vi "svfa_Process FRF.vi"(0 "stimulus signal X [EUx]":waveform(dbl), 1 "response signal Y [EUy]":waveform(dbl), 2 "window":T9=1 items=["None"=0, "Hanning"=1, "Hamming"=2, "Blackman-Harris"=3, "Exact Blackman"=4, "Blackman"=5, "Flat Top"=6, "4 Term B-Harris "=7, "7 Term B-Harris"=8, "Low Sidelobe"=9, "Force - Exponential"=10, "Blackman Nuttall"=11, "Triangle"=30, "Bartlett-Hanning"=31, "Bohman"=32, "Parzen"=33, "Welch"=34, "Kaiser"=60, "Dolph-Chebyshev"=61, "Gaussian"=62], 3 "force/exp settings":T8={"force window [%]"=50.0, "exp window [%]"=10.0} {"exp window [%]" min=0.0 max=100.0 format="%.2f"; "force window [%]" min=0.0 max=100.0 format="%.2f"}, 4 "averaging parameters":T11={"averaging mode"=enum."No averaging", "weighting mode"=enum."Linear", "number of averages"=10, "linear mode"=enum."Auto restart"}, 5 "error in (no error)":errorcluster, 7 "processing control":T10(ring), 9 "FRF mode":enum16{"H1", "H2", "H3"}(ring), 11 "spectrum info in":T1 {"x-axis units" items=["Time (s)"=0, "Frequency-CB (Hz)"=1, "Frequency-CPB (Hz)"=1248, "Frequency-Arbitrary (Hz)"=2357, "Quefrency (s)"=2, "Revolutions (rev)"=3, "Order"=4, "Speed (RPM)"=11, "Speed (rad/s)"=21, "Index"=65535]; "weighting filter" items=["Linear", "A-weighting", "B-weighting", "C-weighting", "ITU-R 468-4", "Dolby", "CCITT", "C-message", "Wb", "Wc", "Wd", "We", "Wf", "Wh", "Wj", "Wk", "Wm", "AES17 20 kHz lowpass", "AES17 40 kHz lowpass", "AES17 20 kHz highpass", "AES17 40 kHz highpass"]; "dB reference [EU]" format="%.2f"; "engineering units" items=["custom..."=0, "V"=1, "A"=21, "C"=30, "pC"=31, "s"=32, "-"=29, "Pa"=2, "N"=20, "g"=3, "m/s^2"=4, "m/s"=5, "m"=6, "mm/s"=12, "mm"=13, "micron/s"=14, "micron"=15, "in/s^2"=7, "in/s"=8, "in"=9, "mil/s"=10, "mil"=11, "rad/s^2"=16, "rad/s"=17, "rad"=18, "deg/s^2"=26, "deg/s"=27, "deg"=28, "RPM"=22, "cycle/s^2"=23, "Hz"=24, "cycle"=25, "strain"=19]; "spectral info"."window" items=["None "=0, "Hanning"=1, "Hamming"=2, "Blackman-Harris"=3, "Exact Blackman"=4, "Blackman"=5, "Flat Top"=6, "4 Term B-Harris "=7, "7 Term B-Harris"=8, "Low Sidelobe"=9, "Force - Exponential"=10, "Gaussian"=62]}) -> (8 "stimulus signal X [EUx]":waveform(dbl), 10 "response signal Y [EUy]":waveform(dbl), 12 "averages completed":dbl format="%.2f", 13 "processing control":T10(ring), 14 "complex frequency response":T7={"f0"=0.0, "df"=1.0, "complex spectrum"=[]} {"complex spectrum" format="%.2f"; "df" format="%.2f"; "f0" format="%.2f"}, 16 "coherence":cluster{"f0":dbl, "df":dbl, "coherence":dbl[]} {"coherence" format="%.2f"; "df" format="%.2f"; "f0" format="%.2f"}, 17 "averaging done":bool, 18 "spectrum info out":T1={"channel name"="", "description"="", "x-axis units"=0, "spectral info"={"spectrum type"=enum."Power [Magnitude^2]", "linear/dB"=enum."linear", "window"=0, "window size"=0, "FFT size"=0}, "engineering units"=0, "custom label"="", "dB reference [EU]"=0.0, "peak units"=enum."rms", "weighting filter"=0, "spectral density?"=FALSE, "unit label"="", "spectrum skewed?"=FALSE, "complimentary spectrum units"=enum."none"} {"x-axis units" items=["Time (s)"=0, "Frequency-CB (Hz)"=1, "Frequency-CPB (Hz)"=1248, "Frequency-Arbitrary (Hz)"=2357, "Quefrency (s)"=2, "Revolutions (rev)"=3, "Order"=4, "Speed (RPM)"=11, "Speed (rad/s)"=21, "Index"=65535]; "weighting filter" items=["Linear", "A-weighting", "B-weighting", "C-weighting", "ITU-R 468-4", "Dolby", "CCITT", "C-message", "Wb", "Wc", "Wd", "We", "Wf", "Wh", "Wj", "Wk", "Wm", "AES17 20 kHz lowpass", "AES17 40 kHz lowpass", "AES17 20 kHz highpass", "AES17 40 kHz highpass"]; "dB reference [EU]" format="%.2f"; "engineering units" items=["custom..."=0, "V"=1, "A"=21, "C"=30, "pC"=31, "s"=32, "-"=29, "Pa"=2, "N"=20, "g"=3, "m/s^2"=4, "m/s"=5, "m"=6, "mm/s"=12, "mm"=13, "micron/s"=14, "micron"=15, "in/s^2"=7, "in/s"=8, "in"=9, "mil/s"=10, "mil"=11, "rad/s^2"=16, "rad/s"=17, "rad"=18, "deg/s^2"=26, "deg/s"=27, "deg"=28, "RPM"=22, "cycle/s^2"=23, "Hz"=24, "cycle"=25, "strain"=19]; "spectral info"."window" items=["None "=0, "Hanning"=1, "Hamming"=2, "Blackman-Harris"=3, "Exact Blackman"=4, "Blackman"=5, "Flat Top"=6, "4 Term B-Harris "=7, "7 Term B-Harris"=8, "Low Sidelobe"=9, "Force - Exponential"=10, "Gaussian"=62]}, 19 "error out":errorcluster)   [LabVIEW 2017]
uses:
  <vilib>/addons/_NISVFA/_Shared subVIs/Controls/svc_Window [Dual FFT].ctl
  <vilib>/addons/_NISVFA/_Shared subVIs/Controls/svc_Spectrum Info.ctl
  <vilib>/addons/_NISVFA/_Shared subVIs/Controls/svc_X-Axis Units.ctl
  <vilib>/addons/_NISVFA/_Shared subVIs/Controls/svc_Spectrum Type.ctl
  <vilib>/addons/_NISVFA/_Shared subVIs/Controls/svc_Engineering Units Text Ring.ctl
  <vilib>/addons/_NISVFA/_Shared subVIs/Controls/svc_Weighting Filter Text Ring.ctl
  <vilib>/addons/_NISVFA/_Shared subVIs/Controls/svc_Complimentary Spectrum Units.ctl
  <vilib>/addons/_NISVFA/_Shared subVIs/Windowing/svfa_Scaled Time Domain Window (1 Ch).vi
  <vilib>/addons/_NISVFA/_Shared subVIs/Spectrum Averaging/svfa_Average Array (complex).vi
  <vilib>/addons/_NISVFA/_Shared subVIs/Spectrum Averaging/svfa_Average Array (real).vi
  <vilib>/addons/_NISVFA/_Shared subVIs/Windowing/svfa_Scaled Time Domain Window (Array).vi
  <vilib>/Analysis/4window.llb/Force Window.vi
  <vilib>/Analysis/4window.llb/Force Window (DBL).vi
  <vilib>/Analysis/4window.llb/Exponential Window.vi
  <vilib>/Analysis/4window.llb/Exponential Window (DBL).vi
  <vilib>/Utility/error.llb/Error Cluster From Error Code.vi
  <vilib>/Analysis/0measdsp.llb/Scaled Time Domain Window.vi
  <vilib>/Analysis/0measdsp.llb/Scaled Time Domain Window (DBL).vi
  <vilib>/addons/_NISVFA/_Spectrum Processing/subVIs/svfa_Spectrum Info Window to windowTd Type Def.vi
  <vilib>/addons/_NISVFA/_Shared subVIs/Common/svc_Window Parameters.vi
  <vilib>/addons/_NISVFA/_Shared subVIs/Common/svc_Get Window Info.vi
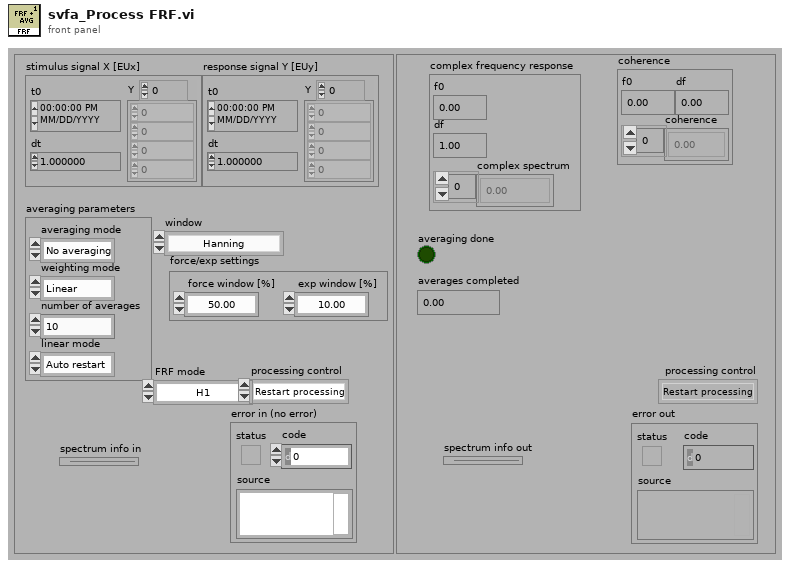
[diagram p1: front panel]
types:
  T1 = typedef "svc_Spectrum Info.ctl" = cluster{"channel name":string, "description":string, "x-axis units":T2, "spectral info":cluster{"spectrum type":T3, "linear/dB":enum16{"linear", "dB"}, "window":u16, "window size":i32, "FFT size":i32}, "engineering units":T4, "custom label":string, "dB reference [EU]":dbl, "peak units":enum16{"rms", "peak", "peak-peak"}, "weighting filter":T5, "spectral density?":bool, "unit label":string, "spectrum skewed?":bool, "complimentary spectrum units":T6}
  T2 = typedef "svc_X-Axis Units.ctl" = u16
  T3 = typedef "svc_Spectrum Type.ctl" = enum16{"FFT Spectrum [complex]", "Amplitude [Magnitude]", "Power [Magnitude^2]", "Cross Spectrum [complex]", "Frequency Response [Complex]"}
  T4 = typedef "svc_Engineering Units Text Ring.ctl" = u16
  T5 = typedef "svc_Weighting Filter Text Ring.ctl" = u16
  T6 = typedef "svc_Complimentary Spectrum Units.ctl" = enum16{"none", "radians", "degrees", "cycles", "imaginary"}
  T7 = cluster{"f0":dbl, "df":dbl, "complex spectrum":cdb[]}
  T8 = cluster{"force window [%]":dbl, "exp window [%]":dbl}
  T9 = typedef "svc_Window [Dual FFT].ctl" = u32
  T10 = enum16{"Restart processing", "Continue processing", "Skip processing"}
  T11 = cluster{"averaging mode":enum16{"No averaging", "Vector averaging", "RMS averaging", "Peak hold"}, "weighting mode":enum16{"Linear", "Exponential"}, "number of averages":u32, "linear mode":enum16{"One shot", "Auto restart"}}
  T12 = enum16{"No averaging", "Vector averaging", "RMS averaging", "Peak hold"}
  T13 = cluster{"f0":dbl, "df":dbl, "complex array":cdb[]}
  T14 = cluster{"complex spectrum":cluster{"f0":dbl, "df":dbl, "complex spectrum":cdb[]}, "spectrum info":T1}
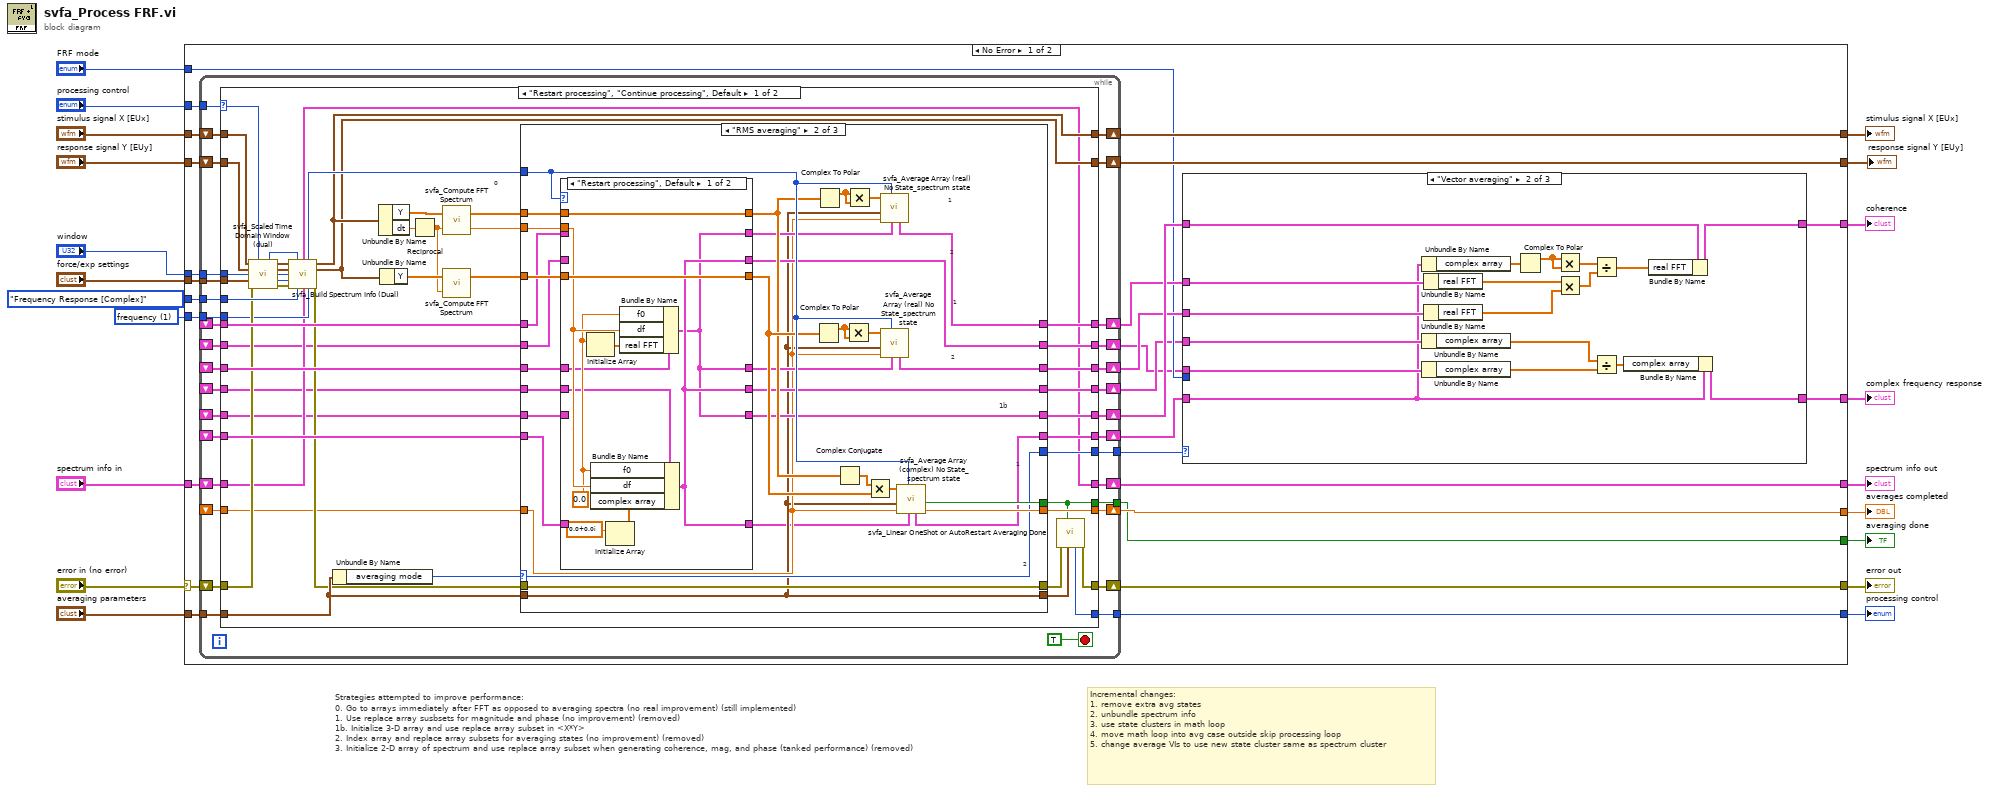
[diagram p0: block diagram]
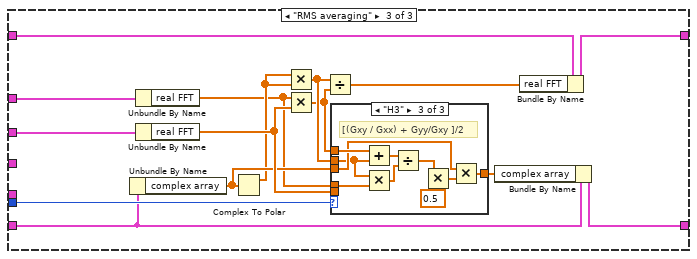
[diagram p3: hidden frame]
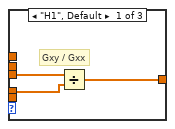
[diagram p4: hidden frame]
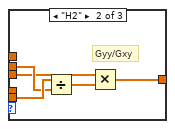
[diagram p5: hidden frame]
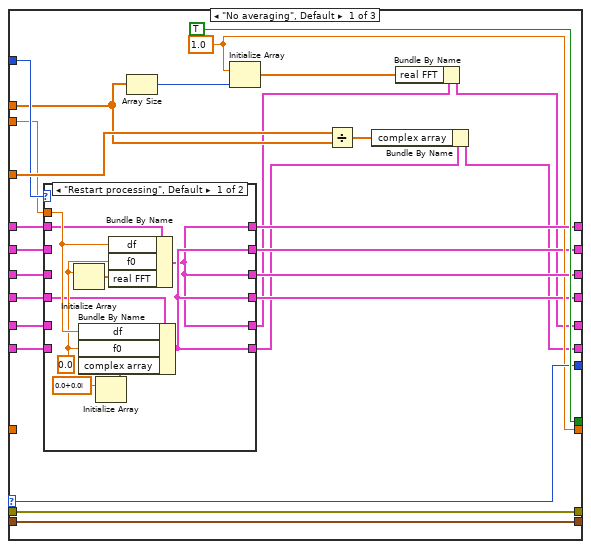
[diagram p6: hidden frame]
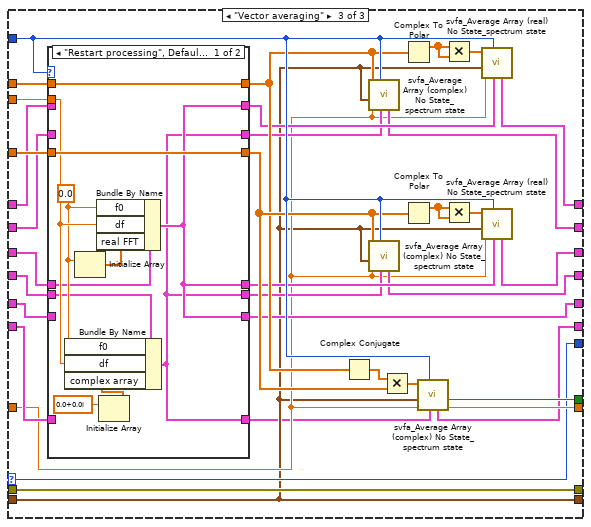
[diagram p9: hidden frame]
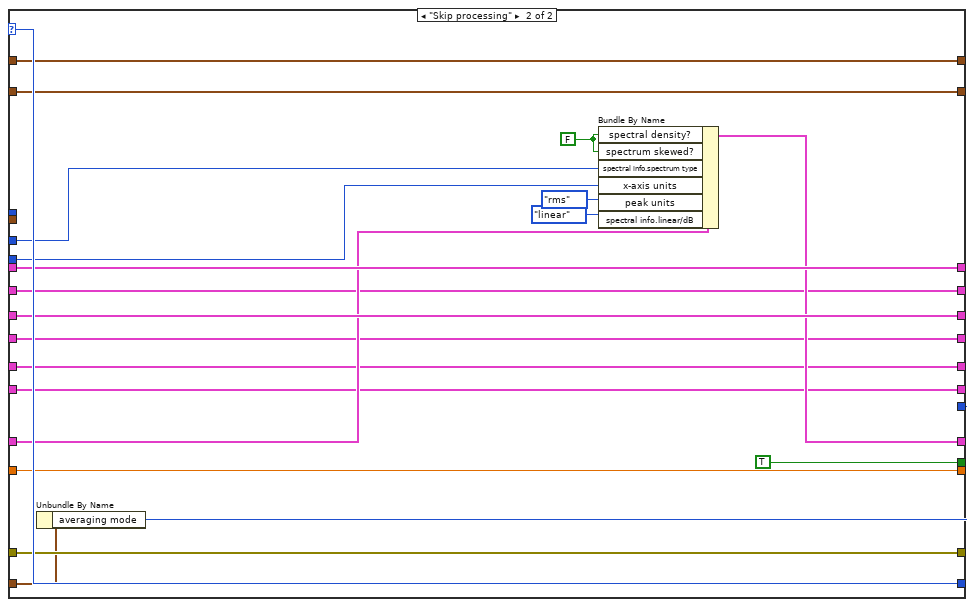
[diagram p11: hidden frame]
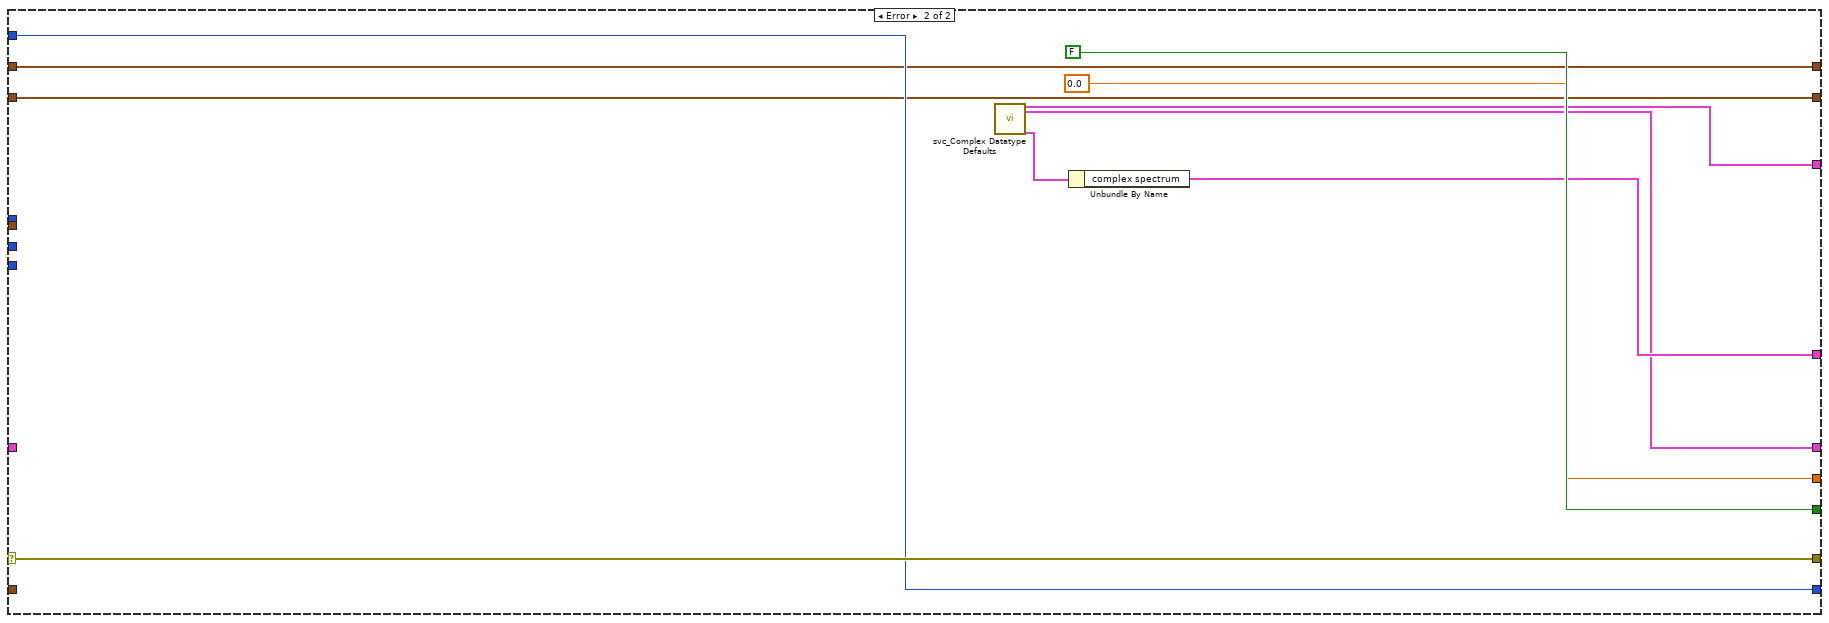
[diagram p12: hidden frame]
diagram:
  w6 = u16 1 items=["time"=0, "frequency"=1, "quefrency"=2, "revolutions"=3, "order"=4, "rpm"=11] ("x-axis units")
  # "Strategies attempted to improve performance:\n0. Go to arrays immediately after FFT as opposed to averaging spectra (no real improvement) (still implemented)\n1. Use replace array susbsets for magnitude and phase (no improvement) (removed)\n1b. Initialize 3-D array and use replace array subset in <X*Y>\n2. Index array and replace array subsets for averaging states (no improvement) (removed)\n3. Initialize 2-D array of spectrum and use replace array subset when generating coherence, mag, and phase (tanked performance) (removed)"
  # "Incremental changes:\n1. remove extra avg states\n2. unbundle spectrum info\n3. use state clusters in math loop\n4. move math loop into avg case outside skip processing loop\n5. change average VIs to use new state cluster same as spectrum cluster"
  n1 = case shown="No Error" "error in (no error)" {
    selector: "error in (no error)" -> [w44 w359]
    tunnel: [w38 w359] -> w20
    tunnel: "averaging parameters" -> [w47 _]
    tunnel: "stimulus signal X [EUx]" -> [w45 w354]
    tunnel: [w32 FALSE ("averaging done")] -> w16
    tunnel: [w46 0.0 ("averages completed")] -> w15
    tunnel: [w22 w352] -> w14
    tunnel: [w23 w350] -> w13
    tunnel: "FRF mode" -> [w26 _]
    tunnel: "processing control" -> [w43 w356]
    tunnel: [w39 w356] -> w10
    tunnel: "response signal Y [EUy]" -> [w42 w353]
    tunnel: "window" -> [w41 _]
    tunnel: "force/exp settings" -> [w40 _]
    tunnel: svc_Spectrum_Type."Frequency Response [Complex]" ("spectrum type") -> [w37 _]
    tunnel: w6 -> [w36 _]
    tunnel: [w35 w351] -> w5
    tunnel: [w34 w354] -> w4
    tunnel: [w33 w353] -> w3
    tunnel: "spectrum info in" -> [w21 _]
    frame No Error {
      n2 = while {
        tunnel: [w124] -> w39
        tunnel: w40 -> [w125]
        tunnel: w41 -> [w126]
        tunnel: w43 -> [w121]
        tunnel: [w130] -> w32
        tunnel: w47 -> [w132]
        shift-right: [w120] -> w28
        shift-left: _ -> [w119]
        shift-right: [w102] -> w31
        shift-left: _ -> [w105]
        shift-right: [w118] -> w29
        shift-left: _ -> [w117]
        tunnel: w37 -> [w116]
        tunnel: w36 -> [w115]
        tunnel: [w112] -> w27
        shift-right: [w111] -> w34
        shift-left: w45 -> [w129]
        shift-right: [w110] -> w33
        shift-left: w42 -> [w127]
        shift-right: [w123] -> w38
        shift-left: w44 -> [w128]
        shift-right: [w113] -> w35
        shift-left: w21 -> [w114]
        shift-right: [w104] -> w24
        shift-left: _ -> [w107]
        shift-right: [w103] -> w25
        shift-left: _ -> [w106]
        shift-right: [w109] -> w30
        shift-left: _ -> [w108]
        shift-right: [w131] -> w46
        shift-left: _ -> [w101]
        stop <- TRUE stop-if-true
        n3 = case shown="\"Restart processing\", \"Continue processing\", Default" w121 {
          selector: w121 -> [w170 w349]
          tunnel: w132 -> [w166 w340]
          tunnel: [w180 w336] -> w131
          tunnel: [w179 TRUE ("averaging done")] -> w130
          tunnel: w128 -> [w152 w347]
          tunnel: w127 -> [w175 w337]
          tunnel: w126 -> [w174 _]
          tunnel: w125 -> [w162 _]
          tunnel: [w171 w349] -> w124
          tunnel: [w167 w347] -> w123
          tunnel: w129 -> [w176 w338]
          tunnel: [w161 w341] -> w109
          tunnel: [w160 w346] -> w120
          tunnel: w108 -> [w159 w341]
          tunnel: w119 -> [w158 w346]
          tunnel: [w157 w345] -> w118
          tunnel: w117 -> [w156 w345]
          tunnel: w116 -> [w155 w329]
          tunnel: w115 -> [w151 w342]
          tunnel: w114 -> [w150 w344]
          tunnel: [w136 w343] -> w113
          tunnel: [w149 w339] -> w112
          tunnel: [w146 w338] -> w111
          tunnel: [w145 w337] -> w110
          tunnel: w107 -> [w144 w335]
          tunnel: w106 -> [w143 w334]
          tunnel: w105 -> [w142 w333]
          tunnel: [w141 w335] -> w104
          tunnel: [w140 w334] -> w103
          tunnel: [w139 w333] -> w102
          tunnel: w101 -> [w138 w336]
          frame "Restart processing", "Continue processing", Default {
            # "0"
            n4 = call <vilib>:"svfa_Scaled Time Domain Window (dual).vi"("Signal in [X]"=w176, "processing control"=w170, "Signal in [Y]"=w175, "window"=w174, "force/exp settings"=w162, "error in (no error)"=w152) -> ("dup processing control"=w169:T10, "Windowed signal [X]"=w178:waveform(dbl), "Windowed signal [Y]"=w177:waveform(dbl), "window"=w173:T9, "window size"=w164:i32, "error out"=w163:errorcluster)  [unwired: 3 in, 1 out]
            n5 = call <vilib>:"svfa_Build Spectrum Info (Dual).vi"("scaled signal  X [EU]"=w178, "processing control"=w169, "scaled signal  Y [EU]"=w177, "window"=w173, "window size"=w164, "error in (no error)"=w163, "spectrum type"=w155, "spectrum info in"=w150, "x-axis units"=w151) -> ("spectrum info out"=w136:T1, "dup processing control"=w168:T10, "dup scaled signal  X [EU]"=w146:waveform(dbl), "dup scaled signal  Y [EU]"=w145:waveform(dbl), "error out"=w147:errorcluster)  [unwired: 2 in]
            n6 = Unbundle By Name(w166) -> ("averaging mode"=w181:T12)
            n7 = Unbundle By Name ("Get Waveform Components")(w146) -> ("Y"=w135:dbl[], "dt"=w134:dbl)
            n8 = Unbundle By Name ("Get Waveform Components")(w145) -> ("Y"=w137:dbl[])
            n9 = Reciprocal(x=w134) -> (1/x=w133:dbl)
            n10 = call <vilib>:"svfa_Compute FFT Spectrum.vi"("sampling frequency [Hz]"=w133, "signal [EU]"=w135) -> ("df [Hz]"=w148:dbl, "FFT spectrum [EUrms]"=w165:cdb[])
            n11 = call <vilib>:"svfa_Compute FFT Spectrum.vi"("sampling frequency [Hz]"=w133, "signal [EU]"=w137) -> ("FFT spectrum [EUrms]"=w154:cdb[])  [unwired: 1 out]
            n12 = case shown="\"RMS averaging\"" w181 {
              selector: w181 -> [w197 w240 w294]
              tunnel: [w205 w239 w293] -> w153
              tunnel: w147 -> [w205 w239 w293]
              tunnel: w166 -> [w206 w231 w283]
              tunnel: [TRUE ("averaging done") w255 w309] -> w179
              tunnel: w168 -> [w203 w253 w307]
              tunnel: [w194 w254 w308] -> w180
              tunnel: [w206 w231 w283] -> w172
              tunnel: w165 -> [w195 w251 w305]
              tunnel: w154 -> [w204 w252 w306]
              tunnel: [w182 w224 w275] -> w161
              tunnel: [w198 w242 w296] -> w160
              tunnel: w159 -> [w200 w246 w301]
              tunnel: w158 -> [w201 w245 w298]
              tunnel: [w199 w243 w297] -> w157
              tunnel: w156 -> [w202 w244 w299]
              tunnel: w148 -> [w196 w241 w295]
              tunnel: [w197 w240 w294] -> w149
              tunnel: w144 -> [w189 w237 w287]
              tunnel: w143 -> [w191 w235 w286]
              tunnel: w142 -> [w192 w233 w285]
              tunnel: [w190 w238 w291] -> w141
              tunnel: [w188 w236 w289] -> w140
              tunnel: [w185 w234 w288] -> w139
              tunnel: w138 -> [_ w232 w284]
              frame "No averaging", Default {
                w194 = 1.0 ("overwrite value")
                n13 = case shown="\"Restart processing\", Default" w203 {
                  tunnel: [w209 w222] -> w199
                  tunnel: w202 -> [w208 w222]
                  tunnel: [w209 w221] -> w198
                  tunnel: w201 -> [_ w221]
                  tunnel: [w210 w220] -> w183
                  tunnel: w200 -> [_ w220]
                  tunnel: w196 -> [w216 _]
                  tunnel: w192 -> [_ w217]
                  tunnel: w191 -> [w211 w218]
                  tunnel: w189 -> [_ w219]
                  tunnel: [w210 w219] -> w190
                  tunnel: [w210 w218] -> w188
                  tunnel: [w209 w217] -> w184
                  frame "Restart processing", Default {
                    w214 = 0.0 ("f0")
                    n14 = Initialize Array(w214) -> (w215:dbl[])  [unwired: 1 in]
                    n15 = Initialize Array(cdb 0.0+0.0i ("element")) -> (w212:cdb[])  [unwired: 1 in]
                    n16 = Bundle By Name(cluster=w211, "df"=w216, "f0"=w214, "complex array"=w212) -> (w210:T13)
                    n17 = Bundle By Name(cluster=w208, "df"=w216, "f0"=w214, "real FFT"=w215) -> (w209:cluster{"f0":dbl, "df":dbl, "real FFT":dbl[]})
                  }
                  frame "Continue processing" {
                  }
                }
                n18 = Array Size(array=w195) -> (size(s)=w186:i32)
                n19 = Initialize Array(w194, w186) -> (w193:dbl[])
                n20 = Divide(x=w204, y=w195) -> (x/y=w187:cdb[])
                n21 = Bundle By Name(cluster=w183, "complex array"=w187) -> (w182:T13)
                n22 = Bundle By Name(cluster=w184, "real FFT"=w193) -> (w185:cluster{"f0":dbl, "df":dbl, "real FFT":dbl[]})
              }
              frame "RMS averaging" {
                # "1"
                # "1b"
                # "2"
                # "2"
                # "2"
                # "1"
                # "1"
                n23 = case shown="\"Restart processing\", Default" w253 {
                  tunnel: w252 -> [w266 w271]
                  tunnel: w251 -> [w264 w274]
                  tunnel: [w266 w271] -> w250
                  tunnel: [w264 w274] -> w249
                  tunnel: [w257 w273] -> w223
                  tunnel: [w256 w272] -> w248
                  tunnel: [w256 w270] -> w247
                  tunnel: w246 -> [_ w273]
                  tunnel: w244 -> [_ w272]
                  tunnel: w245 -> [w259 w270]
                  tunnel: w241 -> [w265 _]
                  tunnel: [w257 w269] -> w238
                  tunnel: w237 -> [_ w269]
                  tunnel: [w257 w268] -> w236
                  tunnel: w235 -> [w258 w268]
                  tunnel: [w256 w267] -> w234
                  tunnel: w233 -> [_ w267]
                  frame "Restart processing", Default {
                    w262 = 0.0 ("f0")
                    n24 = Initialize Array(w262) -> (w263:dbl[])  [unwired: 1 in]
                    n25 = Initialize Array(cdb 0.0+0.0i ("element")) -> (w260:cdb[])  [unwired: 1 in]
                    n26 = Bundle By Name(cluster=w258, "f0"=w262, "df"=w265, "complex array"=w260) -> (w257:T13)
                    n27 = Bundle By Name(cluster=w259, "f0"=w262, "df"=w265, "real FFT"=w263) -> (w256:cluster{"f0":dbl, "df":dbl, "real FFT":dbl[]})
                  }
                  frame "Continue processing", "Skip processing" {
                  }
                }
                n28 = Complex To Polar(r * e^(i*theta)=w250) -> (r=w230:dbl[])  [unwired: 1 out]
                n29 = Complex To Polar(r * e^(i*theta)=w249) -> (r=w228:dbl[])  [unwired: 1 out]
                n30 = Complex Conjugate(1:w249) -> (0:w225:cdb[])
                n31 = Multiply(x=w230, y=w230) -> (x*y=w229:dbl[])
                n32 = Multiply(x=w228, y=w228) -> (x*y=w227:dbl[])
                n33 = Multiply(x=w225, y=w250) -> (x*y=w226:cdb[])
                n34 = call <vilib>:"svfa_Average Array (real) No State_spectrum state.vi"("previous avg real spectrum"=w248, "processing control"=w253, "averages completed"=w232, "averaging parameters"=w231, "array"=w227) -> ("new avg real spectrum"=w243:cluster{"f0":dbl, "df":dbl, "real FFT":dbl[]})  [unwired: 4 in, 2 out]
                n35 = call <vilib>:"svfa_Average Array (real) No State_spectrum state.vi"("previous avg real spectrum"=w247, "processing control"=w253, "averages completed"=w232, "averaging parameters"=w231, "array"=w229) -> ("new avg real spectrum"=w242:cluster{"f0":dbl, "df":dbl, "real FFT":dbl[]})  [unwired: 4 in, 2 out]
                n36 = call <vilib>:"svfa_Average Array (complex) No State_spectrum state.vi"("previous avg complex spectrum"=w223, "processing control"=w253, "averages completed in"=w232, "averaging parameters"=w231, "array"=w226) -> ("averages completed out"=w254:dbl, "averaging done"=w255:bool, "avg complex spectrum"=w224:T13)  [unwired: 4 in]
              }
              frame "Vector averaging" {
                n37 = case shown="\"Restart processing\", Default" w307 {
                  tunnel: w306 -> [w320 w328]
                  tunnel: w305 -> [w318 w327]
                  tunnel: [w320 w328] -> w304
                  tunnel: [w318 w327] -> w303
                  tunnel: [w310 w326] -> w276
                  tunnel: [w311 w325] -> w302
                  tunnel: w301 -> [_ w326]
                  tunnel: w299 -> [_ w325]
                  tunnel: [w311 w324] -> w300
                  tunnel: w298 -> [w313 w324]
                  tunnel: w295 -> [w319 _]
                  tunnel: [w310 w323] -> w292
                  tunnel: [w310 w322] -> w290
                  tunnel: [w311 w321] -> w288
                  tunnel: w287 -> [_ w323]
                  tunnel: w286 -> [w312 w322]
                  tunnel: w285 -> [_ w321]
                  frame "Restart processing", Default {
                    w317 = 0.0 ("f0")
                    n38 = Initialize Array(w317) -> (w316:dbl[])  [unwired: 1 in]
                    n39 = Bundle By Name(cluster=w313, "f0"=w317, "df"=w319, "real FFT"=w316) -> (w311:cluster{"f0":dbl, "df":dbl, "real FFT":dbl[]})
                    n40 = Initialize Array(cdb 0.0+0.0i ("element")) -> (w314:cdb[])  [unwired: 1 in]
                    n41 = Bundle By Name(cluster=w312, "f0"=w317, "df"=w319, "complex array"=w314) -> (w310:T13)
                  }
                  frame "Continue processing", "Skip processing" {
                  }
                }
                n42 = Complex Conjugate(1:w303) -> (0:w278:cdb[])
                n43 = call <vilib>:"svfa_Average Array (complex) No State_spectrum state.vi"("previous avg complex spectrum"=w292, "processing control"=w307, "averages completed in"=w284, "averaging parameters"=w283, "array"=w303) -> ("avg complex spectrum"=w291:T13)  [unwired: 4 in, 2 out]
                n44 = call <vilib>:"svfa_Average Array (complex) No State_spectrum state.vi"("previous avg complex spectrum"=w290, "processing control"=w307, "averages completed in"=w284, "averaging parameters"=w283, "array"=w304) -> ("avg complex spectrum"=w289:T13)  [unwired: 4 in, 2 out]
                n45 = Multiply(x=w278, y=w304) -> (x*y=w277:cdb[])
                n46 = Complex To Polar(r * e^(i*theta)=w303) -> (r=w280:dbl[])  [unwired: 1 out]
                n47 = Complex To Polar(r * e^(i*theta)=w304) -> (r=w282:dbl[])  [unwired: 1 out]
                n48 = call <vilib>:"svfa_Average Array (complex) No State_spectrum state.vi"("previous avg complex spectrum"=w276, "processing control"=w307, "averages completed in"=w284, "averaging parameters"=w283, "array"=w277) -> ("averages completed out"=w308:dbl, "averaging done"=w309:bool, "avg complex spectrum"=w275:T13)  [unwired: 4 in]
                n49 = Multiply(x=w280, y=w280) -> (x*y=w279:dbl[])
                n50 = Multiply(x=w282, y=w282) -> (x*y=w281:dbl[])
                n51 = call <vilib>:"svfa_Average Array (real) No State_spectrum state.vi"("previous avg real spectrum"=w302, "processing control"=w307, "averages completed"=w284, "averaging parameters"=w283, "array"=w279) -> ("new avg real spectrum"=w297:cluster{"f0":dbl, "df":dbl, "real FFT":dbl[]})  [unwired: 4 in, 2 out]
                n52 = call <vilib>:"svfa_Average Array (real) No State_spectrum state.vi"("previous avg real spectrum"=w300, "processing control"=w307, "averages completed"=w284, "averaging parameters"=w283, "array"=w281) -> ("new avg real spectrum"=w296:cluster{"f0":dbl, "df":dbl, "real FFT":dbl[]})  [unwired: 4 in, 2 out]
              }
            }
            n53 = call <vilib>:"svfa_Linear OneShot or AutoRestart Averaging Done.vi"("averaging parameters"=w172, "averaging done"=w179, "error in (no error)"=w153) -> ("error out"=w167:errorcluster, "processing control"=w171:T10)  [unwired: 7 in]
          }
          frame "Skip processing" {
            w331 = FALSE ("spectral density?")
            n54 = Unbundle By Name(w340) -> ("averaging mode"=w339:T12)
            n55 = Bundle By Name(cluster=w344, "spectral density?"=w331, "spectrum skewed?"=w331, "spectral info.spectrum type"=w329, "x-axis units"=w342, "peak units"=enum16{"rms", "peak", "peak-peak"}."rms", "spectral info.linear/dB"=enum16{"linear", "dB"}."linear") -> (w343:T1)
          }
        }
      }
      n56 = case shown="\"Vector averaging\"" w27 {
        tunnel: w30 -> [w48 w53 w69]
        tunnel: w28 -> [_ w67 w81]
        tunnel: w29 -> [_ w66 w82]
        tunnel: [w49 w50 w70] -> w23
        tunnel: [w48 w52 w68] -> w22
        tunnel: w26 -> [_ _ w80]
        tunnel: w31 -> [w49 w51 w71]
        tunnel: w24 -> [_ w65 _]
        tunnel: w25 -> [_ w64 _]
        frame "No averaging", Default {
        }
        frame "Vector averaging" {
          n57 = Unbundle By Name(w53) -> ("complex array"=w60:cdb[])
          n58 = Unbundle By Name(w64) -> ("complex array"=w59:cdb[])
          n59 = Unbundle By Name(w65) -> ("complex array"=w54:cdb[])
          n60 = Unbundle By Name(w66) -> ("real FFT"=w55:dbl[])
          n61 = Unbundle By Name(w67) -> ("real FFT"=w61:dbl[])
          n62 = Complex To Polar(r * e^(i*theta)=w60) -> (r=w56:dbl[])  [unwired: 1 out]
          n63 = Multiply(x=w56, y=w56) -> (x*y=w63:dbl[])
          n64 = Multiply(x=w55, y=w61) -> (x*y=w62:dbl[])
          n65 = Divide(x=w63, y=w62) -> (x/y=w58:dbl[])
          n66 = Divide(x=w59, y=w54) -> (x/y=w57:cdb[])
          n67 = Bundle By Name(cluster=w53, "complex array"=w57) -> (w52:T13)
          n68 = Bundle By Name(cluster=w51, "real FFT"=w58) -> (w50:cluster{"f0":dbl, "df":dbl, "real FFT":dbl[]})
        }
        frame "RMS averaging" {
          n69 = Unbundle By Name(w69) -> ("complex array"=w77:cdb[])
          n70 = Unbundle By Name(w82) -> ("real FFT"=w73:dbl[])
          n71 = Unbundle By Name(w81) -> ("real FFT"=w79:dbl[])
          n72 = Complex To Polar(r * e^(i*theta)=w77) -> (r=w74:dbl[])  [unwired: 1 out]
          n73 = Multiply(x=w74, y=w74) -> (x*y=w75:dbl[])
          n74 = Multiply(x=w73, y=w79) -> (x*y=w72:dbl[])
          n75 = Divide(x=w75, y=w72) -> (x/y=w78:dbl[])
          n76 = case shown="\"H3\"" w80 {
            tunnel: [w85 w86 w98] -> w76
            tunnel: w73 -> [w84 _ w94]
            tunnel: w79 -> [_ w90 _]
            tunnel: w77 -> [w83 w87 w92]
            tunnel: w75 -> [_ w89 w91]
            tunnel: w72 -> [_ _ w97]
            frame "H1", Default {
              # "Gxy / Gxx"
              n77 = Divide(x=w83, y=w84) -> (x/y=w85:cdb[])
            }
            frame "H2" {
              # "Gyy/Gxy"
              n78 = Divide(x=w90, y=w89) -> (x/y=w88:dbl[])
              n79 = Multiply(x=w87, y=w88) -> (x*y=w86:cdb[])
            }
            frame "H3" {
              # "[(Gxy / Gxx) + Gyy/Gxy ]/2"
              n80 = Add(x=w97, y=w91) -> (x+y=w96:dbl[])
              n81 = Multiply(x=w91, y=w94) -> (x*y=w93:dbl[])
              n82 = Divide(x=w96, y=w93) -> (x/y=w95:dbl[])
              n83 = Multiply(x=w95, y=0.5) -> (x*y=w99:dbl[])
              n84 = Multiply(x=w92, y=w99) -> (x*y=w98:cdb[])
            }
          }
          n85 = Bundle By Name(cluster=w69, "complex array"=w76) -> (w68:T13)
          n86 = Bundle By Name(cluster=w71, "real FFT"=w78) -> (w70:cluster{"f0":dbl, "df":dbl, "real FFT":dbl[]})
        }
      }
    }
    frame Error {
      n87 = call <vilib>:"svc_Complex Datatype Defaults.vi"() -> ("empty spectrum"=w350:cluster{"f0":dbl, "df":dbl, "magnitude":dbl[]}, "dead spectrum info"=w351:T1, "complex spectrum"=w355:T14)  [unwired: 11 in, 6 out]
      n88 = Unbundle By Name(w355) -> ("complex spectrum"=w352:T7)
    }
  }
  "error out" <- w20
  "averages completed" <- w15
  "averaging done" <- w16
  "complex frequency response" <- w14
  "coherence" <- w13
  "processing control" <- w10
  "spectrum info out" <- w5
  "stimulus signal X [EUx]" <- w4
  "response signal Y [EUy]" <- w3
